vi "SaveLVlib.vi"(0 "Library in":refnum<vi>, 5 "Library Name":string, 7 "Project Path":path, 11 "error in (no error)":errorcluster) -> (4 "Library out":refnum<vi>, 15 "error out":errorcluster)   [LabVIEW 2016, in "ScriptSubVIs.lvlib"]
doc: "Saves the LV Library inside Tests folder in project location"
uses:
  ScriptSubVIs.lvlib
  <vilib>/SLL Toolkit/SLL File IO/SLL File IO.lvlib
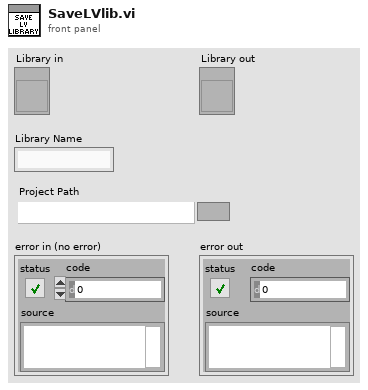
[diagram p1: front panel]
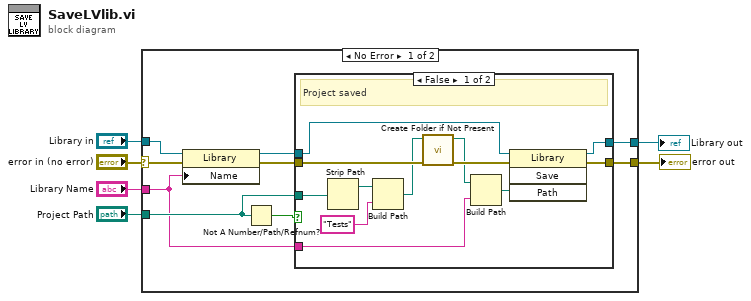
[diagram p0: block diagram]
diagram:
  n1 = case shown="No Error" "error in (no error)" {
    selector: "error in (no error)" -> [w14 w31]
    tunnel: "Library in" -> [w15 w30]
    tunnel: [w12 w31] -> w4
    tunnel: [w10 w30] -> w3
    tunnel: "Project Path" -> [w9 _]
    tunnel: "Library Name" -> [w8 _]
    frame No Error {
      n2 = property class="Library"(reference=w15, error in=w14, "Name"=w8) -> (reference out=w11:refnum<vi>, error out=w7:errorcluster)
      n3 = Not A Number/Path/Refnum?(number/path/refnum=w9) -> (NaN/Path/Refnum?=w13:bool)
      n4 = case shown="False" w13 {
        tunnel: w7 -> [w21 w29]
        tunnel: [w25 w29] -> w12
        tunnel: w11 -> [w27 w28]
        tunnel: [w26 w28] -> w10
        tunnel: w9 -> [w24 _]
        tunnel: w8 -> [w16 _]
        frame False {
          # "Project saved"
          n5 = Strip Path(path=w24) -> (stripped path=w23:path)  [unwired: 1 out]
          n6 = Build Path(base path=w23, name or relative path="Tests" ("string")) -> (appended path=w19:path)
          n7 = call <vilib>:"Create Folder if Not Present.vi"("error in (no error)"=w21, "Path"=w19) -> ("error out"=w20:errorcluster, "Path out"=w17:path)  [unwired: 8 in]
          n8 = Build Path(base path=w17, name or relative path=w16) -> (appended path=w18:path)
          n9 = invoke class="Library" method="Save"(reference=w27, error in=w20, "Path"=w18) -> (reference out=w26:refnum<vi>, error out=w25:errorcluster)  [unwired: 1 in, 2 out]
        }
        frame True {
          # "Project not saved"
        }
      }
    }
    frame Error {
    }
  }
  "Library out" <- w3
  "error out" <- w4
